vi "PQtransaction Status.vi"(8 "error in (no error)":errorcluster, 11 "conn":u64) -> (0 "error out":errorcluster, 2 "transactionstatus":i64, 3 "conn_out":u64)   [LabVIEW 2019, in "libpqlv64.lvlib"]
doc: "Returns the current in-transaction status of the server.\n\nPGTransactionStatusType PQtransactionStatus(const PGconn *conn);\n\nThe status can be PQTRANS_IDLE (currently idle), PQTRANS_ACTIVE (a command is in progress), PQTRANS_INTRANS (idle, in a valid transaction block), or PQTRANS_INERROR (idle, in a failed transaction block). PQTRANS_UNKNOWN is reported if the connection is bad. PQTRANS_ACTIVE is reported only when a query has been sent to the server and not yet completed."
uses:
  libpqlv64.lvlib
  libpq.dll
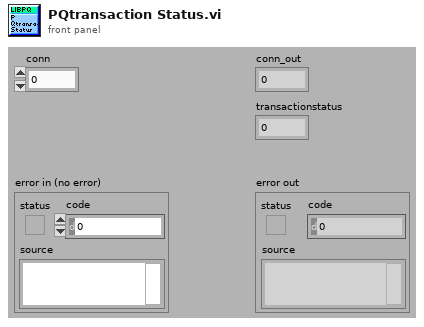
[diagram p1: front panel]
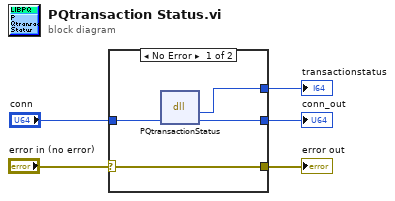
[diagram p0: block diagram]
diagram:
  n1 = case shown="No Error" "error in (no error)" {
    selector: "error in (no error)" -> [w9 w11]
    tunnel: [w9 w11] -> w4
    tunnel: [w8 _] -> w1
    tunnel: "conn" -> [w7 w10]
    tunnel: [w6 w10] -> w2
    frame No Error {
      n2 = dll-call lib="libpq.*" fn="PQtransactionStatus"("conn"=w7) -> ("transactionstatus"=w8:i64, "conn"=w6:u64)  [unwired: 3 in, 2 out]
    }
    frame Error {
    }
  }
  "error out" <- w4
  "conn_out" <- w2
  "transactionstatus" <- w1
